vi "DaNIDemoVI_gpc.vi"() -> ()   [LabVIEW 2016]
uses:
  <vilib>/userdefined/High Color/nirio_resource_hc.ctl
  <vilib>/Analysis/Matrix/Datatypes/RealMatrix.ctl
  <vilib>/Analysis/2dsp.llb/1D Convolution (DBL).vi
  <vilib>/Analysis/7linalg.llb/Real Transpose Matrix.vi
  <vilib>/Analysis/Matrix/Numeric/Conversions/Array To Matrix - RA.vi
  <vilib>/Analysis/Matrix/Numeric/Conversions/Array To Matrix - RA2.vi
  <vilib>/Analysis/7linalg.llb/Create Special Real Matrix.vi
  <vilib>/Analysis/baseanly.llb/Real Inverse Matrix.vi
  <vilib>/Analysis/Matrix/Numeric/Multiply/Multiply - RM,RM.vi
  <vilib>/Analysis/Matrix/Numeric/Add/Add - RM,RM.vi
  <vilib>/Analysis/Matrix/Numeric/Subtract/Subtract - RM,RM.vi
  <vilib>/Analysis/NI_AALPro.lvlib
  <vilib>/Analysis/NI_AALBase.lvlib
  <vilib>/Analysis/Matrix/NI_Matrix.lvlib
panel:
  out "m":i32
  out "n":i32
  in  "B":dbl[](array[numeric])
  in  "A":dbl[](array[numeric])
  out "du term":T1
  out "y term":T1
  out "current setpoint":dbl
  out "r term":T1
  out "Matrix for y":T1
  out "Matrix for du":T1
  out "Matrix for r":T1
  in  "lamda":i32
  in  "Horizon":i32
  out "Q":T1
  out "p":T1
  out "H":T1
  out "Waveform Chart 2":dbl(graph)
  out "Waveform Chart":dbl(graph)
  in  "Mode Select":T2(ring)
  in  "IP Adress":T3="rio://169.254.0.1/RIO0"
  out "Distance Measured (m)":dbl
  in  "Servomotor Angle Offset (Degrees)":dbl
  in  "Servomotor Angle (Degrees)":dbl
  out "Rad/s Right":dbl
  out "Rad/s Left":dbl
  in  "dt (ms)":u32=50
  out "Right Motor Voltage Percentage In (-1 to 1)":dbl min=-1.0 max=1.0 step=0.01
  in  "Left Motor Voltage Percentage In (-1 to 1)":dbl min=-1.0 max=1.0 step=0.01
  in  "stop":bool
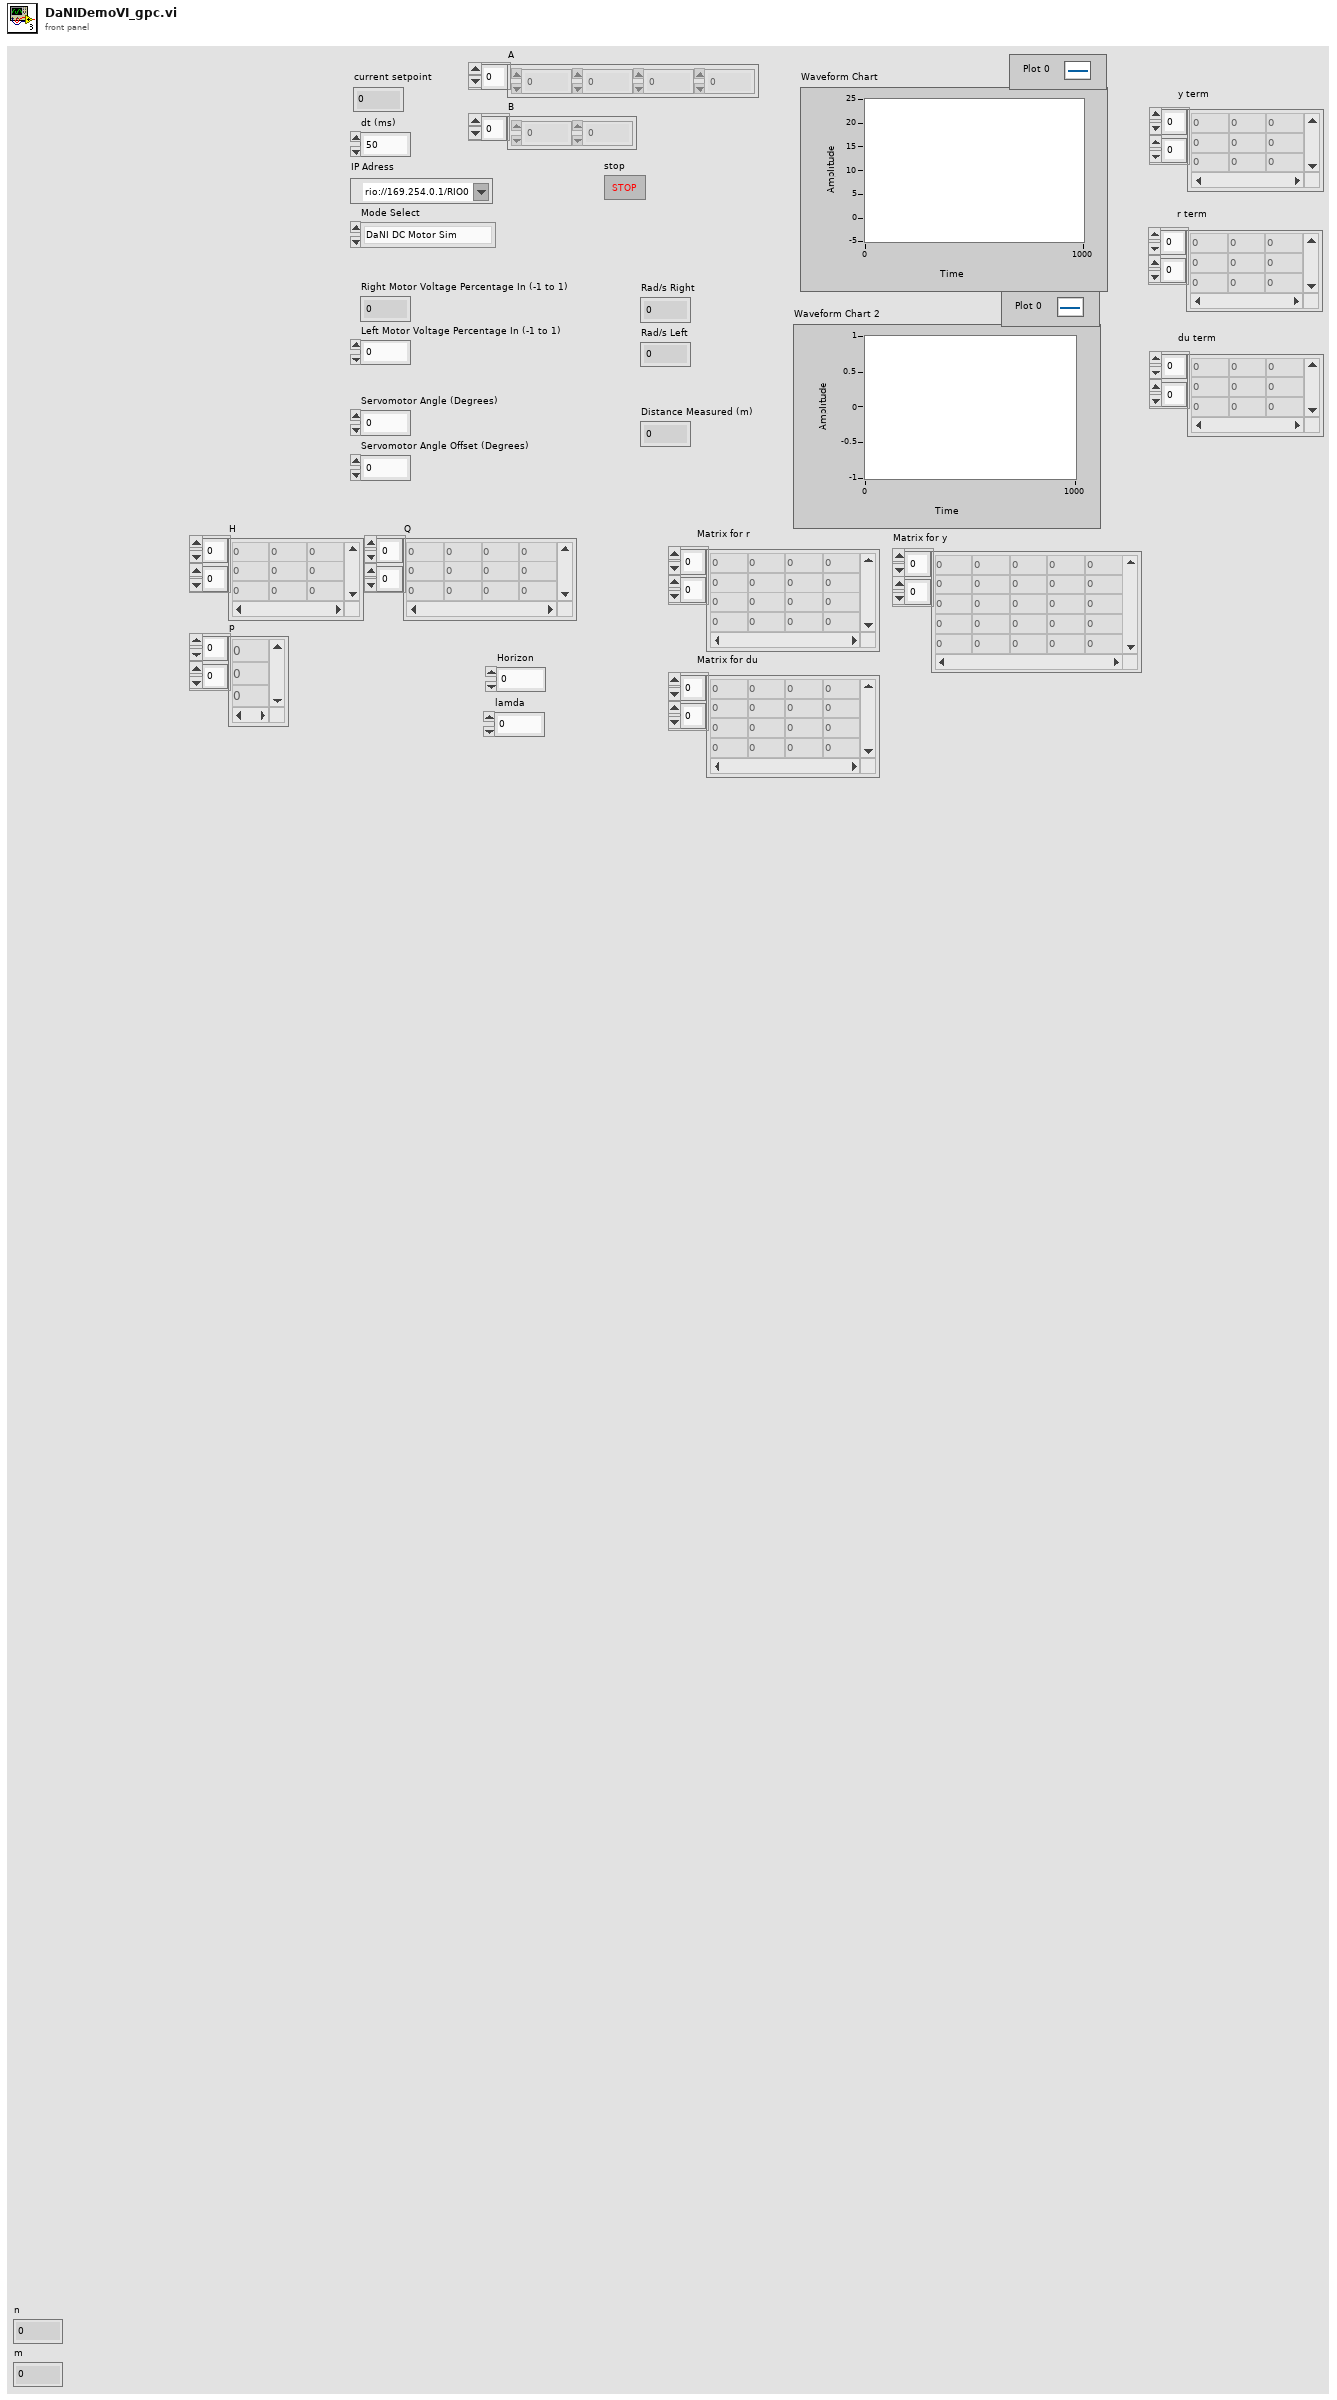
[diagram p1: front panel]
types:
  T1 = typedef "NI_Matrix.lvlib/RealMatrix.ctl" = dbl[][]
  T2 = enum16{"DaNI DC Motor Sim", "DaNI Simulation", "DaNI Robot"}
  T3 = typedef "nirio_resource_hc.ctl" = tag
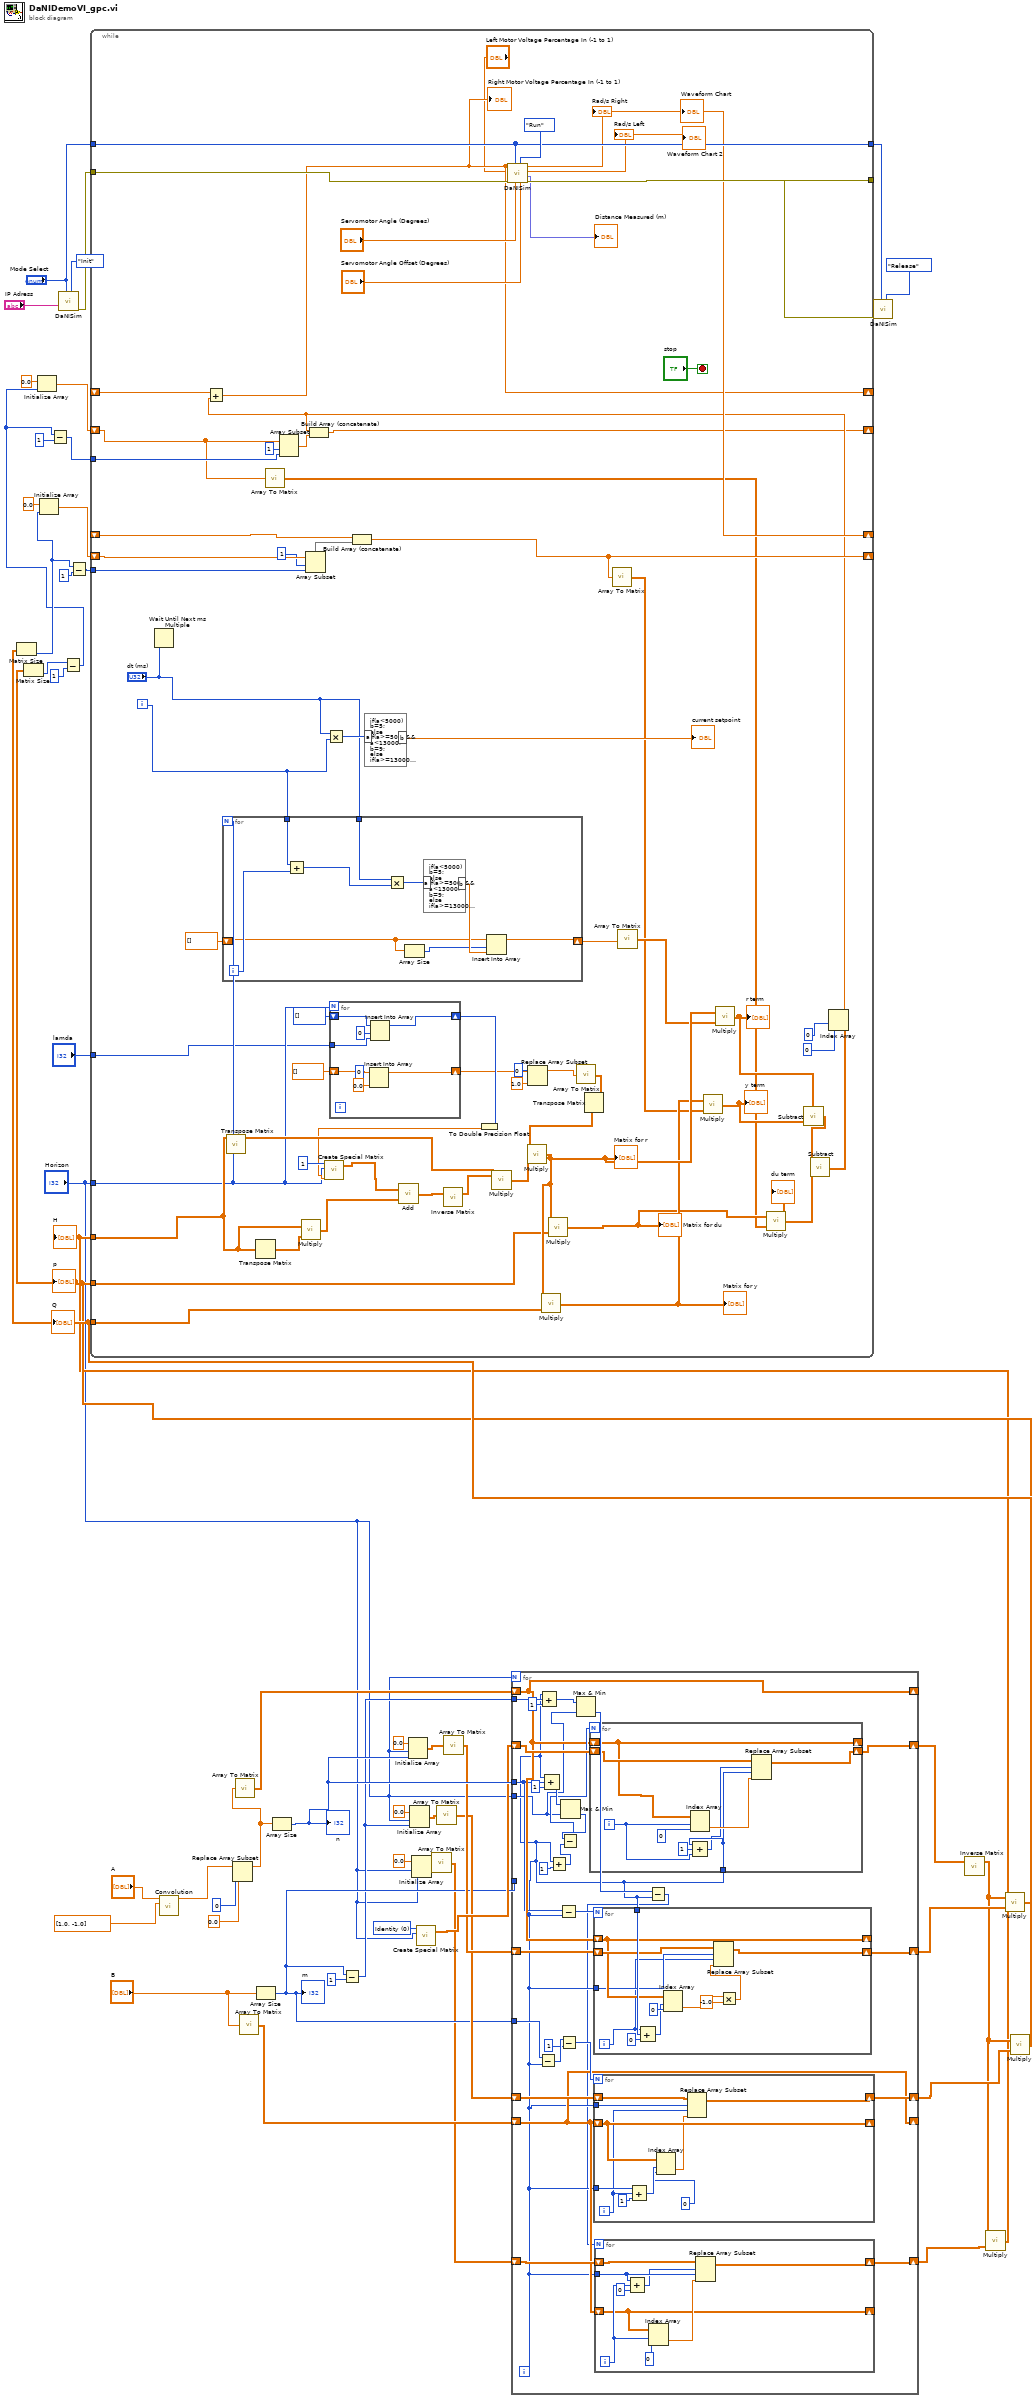
[diagram p0: block diagram]
diagram:
  w25 = 0 items=["Identity", "Diagonal", "Toeplitz", "Vandermonde", "Companion", "Hankel", "Hadamard", "Wilkinson", "Hilbert", "Inverse Hilbert", "Rosser", "Pascal"] ("matrix type")
  n1 = call "DaNISim.vi"("Action"=enum16{"Init", "Run", "Release"}."Init", "Mode Select"="Mode Select", "IP Adress"="IP Adress") -> ("error out"=w51:errorcluster)  [unwired: 5 in, 3 out]
  n2 = call-poly <vilib>:"Convolution.vi"("Y"=dbl[] [1.0, -1.0] ("A 2"), "X"="A") -> ("X * Y"=w31:dbl[])  [unwired: 8 in, 1 out]
  n3 = Replace Array Subset(array=w31, new element=0.0 ("new element/subarray"), index=0) -> (w21:dbl[])
  n4 = call-poly <vilib>:"Array To Matrix.vi"("Real 1D Array"=w21) -> ("Real Matrix (Column Vector)"=w20:T1)
  n5 = call-poly <vilib>:"Array To Matrix.vi"("Real 1D Array"="B") -> ("Real Matrix (Column Vector)"=w13:T1)
  n6 = Array Size(array="B") -> (size(s)=w12:i32)
  "m" <- w12
  n7 = Array Size(array=w21) -> (size(s)=w18:i32)
  "n" <- w18
  n8 = Subtract(x=w12, y=1) -> (x-y=w10:i32)
  n9 = Initialize Array(0.0 ("element"), "Horizon", w18) -> (w24:dbl[][])
  n10 = Initialize Array(0.0 ("element"), "Horizon", w10) -> (w23:dbl[][])
  n11 = Initialize Array(0.0 ("element"), "Horizon", "Horizon") -> (w22:dbl[][])
  n12 = call-poly <vilib>:"Create Special Matrix.vi"("matrix type"=w25, "matrix size"="Horizon") -> ("Special Matrix"=w17:T1)  [unwired: 3 in, 1 out]
  n13 = call-poly <vilib>:"Array To Matrix.vi"("Real 2D Array"=w22) -> ("Real Matrix"=w11:T1)
  n14 = call-poly <vilib>:"Array To Matrix.vi"("Real 2D Array"=w23) -> ("Real Matrix"=w15:T1)
  n15 = call-poly <vilib>:"Array To Matrix.vi"("Real 2D Array"=w24) -> ("Real Matrix"=w16:T1)
  n16 = for {
    N: "Horizon" -> [_]
    shift-right: [w81] -> w9
    shift-left: w17 -> [w82]
    shift-right: [w72] -> _
    shift-left: w20 -> [w72]
    tunnel: w12 -> [_]
    tunnel: w18 -> [w71]
    tunnel: "Horizon" -> [w60]
    shift-right: [w73] -> w8
    shift-left: w16 -> [w74]
    shift-right: [w68] -> w7
    shift-left: w15 -> [w69]
    shift-right: [w61] -> _
    shift-left: w13 -> [w61]
    tunnel: w12 -> [w67]
    shift-right: [w62] -> w6
    shift-left: w11 -> [w63]
    tunnel: w10 -> [w58]
    i -> [w55]
    n17 = Subtract(x=w67, y=w55) -> (x-y=w66:i32)
    n18 = Compound Arithmetic op=ADD(w55, w58, 1 ("value")) -> (w59:i32)
    n19 = Compound Arithmetic op=ADD(w55, w71, 1 ("value")) -> (w79:i32)
    n20 = Add(x=w55, y=1) -> (x+y=w76:i32)
    n21 = Subtract(x=w71, y=w55) -> (x-y=w70:i32)
    n22 = Subtract(x=w66, y=1) -> (x-y=w64:i32)
    n23 = Max & Min(x=w79, y=w60) -> (min(x,y)=w78:i32)  [unwired: 1 out]
    n24 = Subtract(x=w78, y=w76) -> (x-y=w75:i32)
    n25 = Max & Min(x=w59, y=w60) -> (min(x,y)=w56:i32)  [unwired: 1 out]
    n26 = for {
      N: w75 -> [_]
      shift-right: [w121] -> w81
      shift-left: w82 -> [w122]
      tunnel: w55 -> [w117]
      shift-right: [w120] -> _
      shift-left: w72 -> [w120]
      i -> [w115]
      n27 = Index Array(array=w120, index (row)=w115, index (col)=0 ("index (row)")) -> (element=w118:dbl)
      n28 = Compound Arithmetic op=ADD(w117, 1 ("value"), w115) -> (w114:i32)
      n29 = Replace Array Subset(array=w122, new element=w118, index (row)=w114, index (col)=w117) -> (w121:T1)
    }
    n30 = for {
      N: w70 -> [_]
      shift-right: [w108] -> w73
      shift-left: w74 -> [w109]
      shift-right: [w107] -> _
      shift-left: w72 -> [w107]
      tunnel: w55 -> [w112]
      tunnel: w55 -> [w106]
      i -> [w105]
      n31 = Compound Arithmetic op=ADD(w105, w112, 0 ("value")) -> (w110:i32)
      n32 = Index Array(array=w107, index (row)=w110, index (col)=0) -> (element=w103:dbl)
      n33 = Multiply(x=w103, y=-1.0) -> (x*y=w102:dbl)
      n34 = Replace Array Subset(array=w109, new element=w102, index (row)=w106, index (col)=w105) -> (w108:T1)
    }
    n35 = for {
      N: w64 -> [_]
      shift-right: [w99] -> w68
      shift-left: w69 -> [w100]
      shift-right: [w101] -> _
      shift-left: w61 -> [w101]
      tunnel: w55 -> [w97]
      tunnel: w55 -> [w95]
      i -> [w94]
      n36 = Compound Arithmetic op=ADD(w97, w94, 1 ("value")) -> (w93:i32)
      n37 = Index Array(array=w101, index (row)=w93, index (col)=0 ("index (row)")) -> (element=w96:dbl)
      n38 = Replace Array Subset(array=w100, new element=w96, index (row)=w95, index (col)=w94) -> (w99:T1)
    }
    n39 = Subtract(x=w56, y=w55) -> (x-y=w54:i32)
    n40 = for {
      N: w54 -> [_]
      shift-right: [w90] -> w62
      shift-left: w63 -> [w91]
      shift-right: [w83] -> _
      shift-left: w61 -> [w83]
      tunnel: w55 -> [w87]
      i -> [w86]
      n41 = Compound Arithmetic op=ADD(w87, w86, 0 ("value")) -> (w84:i32)
      n42 = Index Array(array=w83, index (row)=w86, index (col)=0) -> (element=w88:dbl)
      n43 = Replace Array Subset(array=w91, new element=w88, index (row)=w84, index (col)=w87) -> (w90:T1)
    }
  }
  n44 = call-poly <vilib>:"Inverse Matrix.vi"("Input Matrix"=w9) -> ("Inverse Matrix"=w5:T1)  [unwired: 1 in, 1 out]
  n45 = call-poly <vilib>:"Multiply.vi"("Real Matrix B"=w6, "Real Matrix A"=w5) -> ("A * B"=w2:T1)
  "H" <- w2
  n46 = call-poly <vilib>:"Multiply.vi"("Real Matrix B"=w8, "Real Matrix A"=w5) -> ("A * B"=w4:T1)
  "Q" <- w4
  n47 = Matrix Size(0:w4) -> (2:w38:i32)  [unwired: 1 out]
  n48 = Initialize Array(0.0 ("element"), w38) -> (w44:dbl[])
  n49 = Subtract(x=w38, y=1) -> (x-y=w37:i32)
  n50 = call-poly <vilib>:"Multiply.vi"("Real Matrix B"=w7, "Real Matrix A"=w5) -> ("A * B"=w3:T1)
  "p" <- w3
  n51 = Matrix Size(0:w3) -> (2:w42:i32)  [unwired: 1 out]
  n52 = Subtract(x=w42, y=1) -> (x-y=w36:i32)
  n53 = Initialize Array(0.0 ("element"), w36) -> (w40:dbl[])
  n54 = Subtract(x=w36, y=1) -> (x-y=w34:i32)
  n55 = while {
    tunnel: w51 -> [w188]
    tunnel: "Mode Select" -> [w182]
    tunnel: [w186] -> w49
    tunnel: [w182] -> w47
    shift-right: [w154] -> _
    shift-left: _ -> [w147]
    tunnel: w4 -> [w153]
    tunnel: w3 -> [w152]
    tunnel: w2 -> [w151]
    tunnel: "Horizon" -> [w150]
    tunnel: "lamda" -> [w149]
    shift-right: [w143] -> _
    shift-left: w44 -> [w146]
    shift-right: [w124] -> _
    shift-left: _ -> [w135]
    shift-right: [w129] -> _
    shift-left: w40 -> [w127]
    tunnel: w37 -> [w133]
    tunnel: w34 -> [w132]
    i -> [w179]
    stop <- "stop" stop-if-true
    n56 = Wait Until Next ms Multiple(millisecond multiple="dt (ms)") -> ()  [unwired: 1 out]
    n57 = for {
      N: w150 -> [_]
      tunnel: w179 -> [w206]
      tunnel: "dt (ms)" -> [w203]
      shift-right: [w200] -> w157
      shift-left: dbl[] [] -> [w199]
      i -> [w205]
      n58 = Add(x=w206, y=w205) -> (x+y=w204:i32)
      n59 = Multiply(x=w203, y=w204) -> (x*y=w202:u32)
      n60 = Array Size(array=w199) -> (size(s)=w198:i32)
      n61 = formula code="if(a<5000)\nb=5;\nelse \nif(a>=5000&&a<13000)\nb=9;\nelse\nif(a>=13000&&a<18000)\nb=13;\nelse\nif(a>=18000&&a<23000)\nb=7;\nelse\nif(a>=23000&&a<33000)\nb=-8;\nelse\nif(a>=33000)\nb=0;"("a"=w202) -> ("b"=w201:dbl)
      n62 = Insert Into Array(array=w199, index=w198, new element=w201) -> (w200:dbl[])
    }
    n63 = call-poly <vilib>:"Transpose Matrix.vi"("Input Matrix"=w151) -> ("Matrix Transpose"=w170:T1)  [unwired: 9 in, 1 out]
    n64 = Transpose Matrix(1:w151) -> (0:w175:T1)
    n65 = call-poly <vilib>:"Array To Matrix.vi"("Real 1D Array"=w127) -> ("Real Matrix (Column Vector)"=w126:T1)
    n66 = Array Subset(array=w127, index=1, length=w132) -> (w131:dbl[])
    n67 = call-poly <vilib>:"Multiply.vi"("Real Matrix B"=w175, "Real Matrix A"=w151) -> ("A * B"=w174:T1)
    n68 = Array Subset(array=w146, index=1, length=w133) -> (w148:dbl[])
    n69 = Multiply(x="dt (ms)", y=w179) -> (x*y=w180:u32)
    n70 = for {
      N: w150 -> [_]
      shift-right: [w197] -> w169
      shift-left: i32[] [] -> [w196]
      tunnel: w149 -> [w190]
      shift-right: [w193] -> w166
      shift-left: dbl[] [] -> [w194]
      n71 = Insert Into Array(array=w194, index=0, new element=0.0 ("new element/subarray")) -> (w193:dbl[])
      n72 = Insert Into Array(array=w196, index=0, new element=w190) -> (w197:i32[])
    }
    n73 = Build Array (concatenate)(w147, w148) -> (w143:dbl[])
    n74 = formula code="if(a<5000)\nb=5;\nelse \nif(a>=5000&&a<13000)\nb=9;\nelse\nif(a>=13000&&a<18000)\nb=13;\nelse\nif(a>=18000&&a<23000)\nb=7;\nelse\nif(a>=23000&&a<33000)\nb=-8;\nelse\nif(a>=33000)\nb=0;"("a"=w180) -> ("b"=→"current setpoint":dbl)
    n75 = To Double Precision Float(number=w169) -> (double precision float=w168:dbl[])
    n76 = call-poly <vilib>:"Create Special Matrix.vi"("matrix type"=1 ("matrix size"), "matrix size"=w150, "Input Vector1"=w168) -> ("Special Matrix"=w173:T1)  [unwired: 2 in, 1 out]
    n77 = call-poly <vilib>:"Add.vi"("Real Matrix B"=w174, "Real Matrix A"=w173) -> ("A + B"=w176:T1)
    n78 = call-poly <vilib>:"Inverse Matrix.vi"("Input Matrix"=w176) -> ("Inverse Matrix"=w171:T1)  [unwired: 1 in, 1 out]
    n79 = call-poly <vilib>:"Multiply.vi"("Real Matrix B"=w170, "Real Matrix A"=w171) -> ("A * B"=w163:T1)
    n80 = Replace Array Subset(array=w166, new element=1.0 ("new element/subarray"), index=0) -> (w162:dbl[])
    n81 = call-poly <vilib>:"Array To Matrix.vi"("Real 1D Array"=w162) -> ("Real Matrix (Column Vector)"=w160:T1)
    n82 = Transpose Matrix(1:w160) -> (0:w161:T1)
    n83 = call-poly <vilib>:"Multiply.vi"("Real Matrix B"=w163, "Real Matrix A"=w161) -> ("A * B"=w158:T1)
    "Matrix for r" <- w158
    n84 = call-poly <vilib>:"Multiply.vi"("Real Matrix B"=w153, "Real Matrix A"=w158) -> ("A * B"=w144:T1)
    "Matrix for y" <- w144
    n85 = call-poly <vilib>:"Multiply.vi"("Real Matrix B"=w152, "Real Matrix A"=w158) -> ("A * B"=w128:T1)
    "Matrix for du" <- w128
    n86 = call-poly <vilib>:"Array To Matrix.vi"("Real 1D Array"=w143) -> ("Real Matrix (Column Vector)"=w142:T1)
    n87 = call-poly <vilib>:"Array To Matrix.vi"("Real 1D Array"=w157) -> ("Real Matrix (Column Vector)"=w156:T1)
    n88 = call-poly <vilib>:"Multiply.vi"("Real Matrix B"=w142, "Real Matrix A"=w144) -> ("A * B"=w140:T1)
    "y term" <- w140
    n89 = call-poly <vilib>:"Multiply.vi"("Real Matrix B"=w156, "Real Matrix A"=w158) -> ("A * B"=w141:T1)
    "r term" <- w141
    n90 = call-poly <vilib>:"Multiply.vi"("Real Matrix B"=w126, "Real Matrix A"=w128) -> ("A * B"=w125:T1)
    "du term" <- w125
    n91 = call-poly <vilib>:"Subtract.vi"("Real Matrix B"=w140, "Real Matrix A"=w141) -> ("A - B"=w139:T1)
    n92 = call-poly <vilib>:"Subtract.vi"("Real Matrix B"=w125, "Real Matrix A"=w139) -> ("A - B"=w138:T1)
    n93 = Index Array(array=w138, index (row)=0 ("disabled index (row)"), index (col)=0 ("disabled index (col)")) -> (element=w130:dbl)
    n94 = Add(x=w135, y=w130) -> (x+y=w124:dbl)
    "Right Motor Voltage Percentage In (-1 to 1)" <- w124
    n95 = Build Array (concatenate)(w130, w131) -> (w129:dbl[])
    n96 = call "DaNISim.vi"("Sonar offset angle"="Servomotor Angle Offset (Degrees)", "Action"=enum16{"Init", "Run", "Release"}."Run", "Sonar angle"="Servomotor Angle (Degrees)", "Mode Select"=w182, "error in (no error)"=w188, "Ul"="Left Motor Voltage Percentage In (-1 to 1)", "Ur"=w124) -> ("error out"=w186:errorcluster, "Sonar distance"=→"Distance Measured (m)":fxp<+,32,8>, "OmegaL"=→"Rad/s Left" →"Waveform Chart 2":dbl, "OmegaR"=w154:dbl)  [unwired: 1 in]
    "Rad/s Right" <- w154
    "Waveform Chart" <- w154
  }
  n97 = call "DaNISim.vi"("Action"=enum16{"Init", "Run", "Release"}."Release", "Mode Select"=w47, "error in (no error)"=w49) -> ()  [unwired: 5 in, 4 out]
